vi "FlatToRichcif_templateplugin_Numeric.vi"(5 "OutputClusterType":T1, 11 "InputCluster":T2) -> (3 "OutputCluster":T1)   [LabVIEW 2021, in "CIFTemplatePlugin_server.lvlib"]
uses:
  CIFTemplatePlugin_server.lvlib
  cif_templateplugin_Numeric_Flat.ctl
  cif_templateplugin_Numeric.ctl
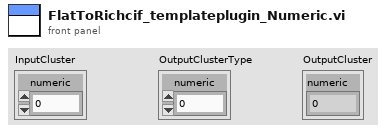
[diagram p1: front panel]
types:
  T1 = typedef "CIFTemplatePlugin_server.lvlib/cif_templateplugin_Numeric.ctl" = cluster{"numeric":i32}
  T2 = typedef "CIFTemplatePlugin_server.lvlib/cif_templateplugin_Numeric_Flat.ctl" = cluster{"numeric":i32}
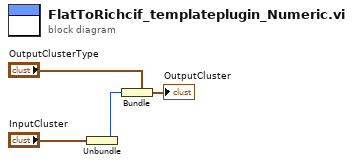
[diagram p0: block diagram]
diagram:
  n1 = Unbundle "Unbundle"("InputCluster") -> ("numeric"=w1:i32)
  n2 = Bundle "Bundle"(cluster="OutputClusterType", "numeric"=w1) -> (→"OutputCluster":T1)
